vi "Read Wait.vi"(0 "Sensor Channel":i32, 2 "Desired Value":bool, 3 "error in (no error)":errorcluster) -> (10 "error out":errorcluster)   [LabVIEW 2016]
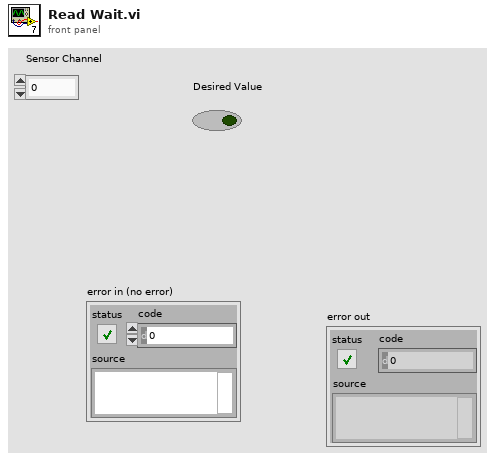
[diagram p1: front panel]
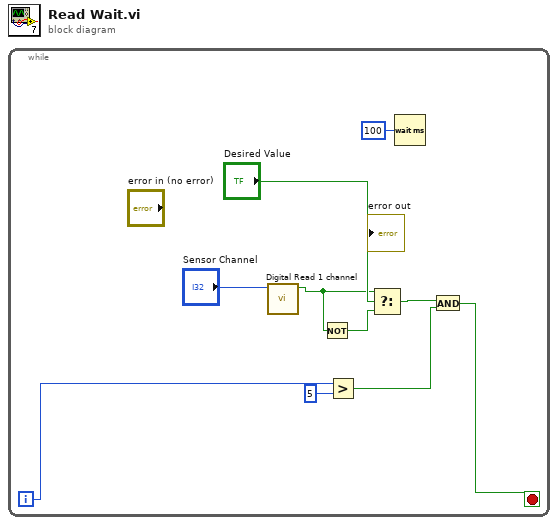
[diagram p0: block diagram]
diagram:
  n1 = while {
    i -> [w5]
    stop <- w3 stop-if-true
    n2 = call "Digital Read 1 channel.vi"("Sensor Channel"="Sensor Channel") -> ("Sensor Value"=w8:bool)  [unwired: 9 in, 1 out]
    n3 = Not(x=w8) -> (.not. x?=w7:bool)
    n4 = Greater?(x=w5, y=5) -> (0:w1:bool)
    n5 = Select(t=w8, s="Desired Value", f=w7) -> (s? t:f=w2:bool)
    n6 = Wait (ms)(milliseconds to wait=u32 100) -> ()  [unwired: 1 out]
    n7 = And(x=w2, y=w1) -> (x .and. y?=w3:bool)
  }
